vi "Find Minima and Walls.vi"() -> (3 "Low Points":cluster{i32, i32}[](array[cluster]), 5 "Wall":bool[][](array[boolean]))   [LabVIEW 2020]
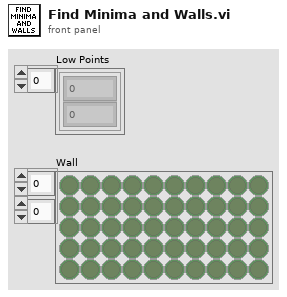
[diagram p1: front panel]
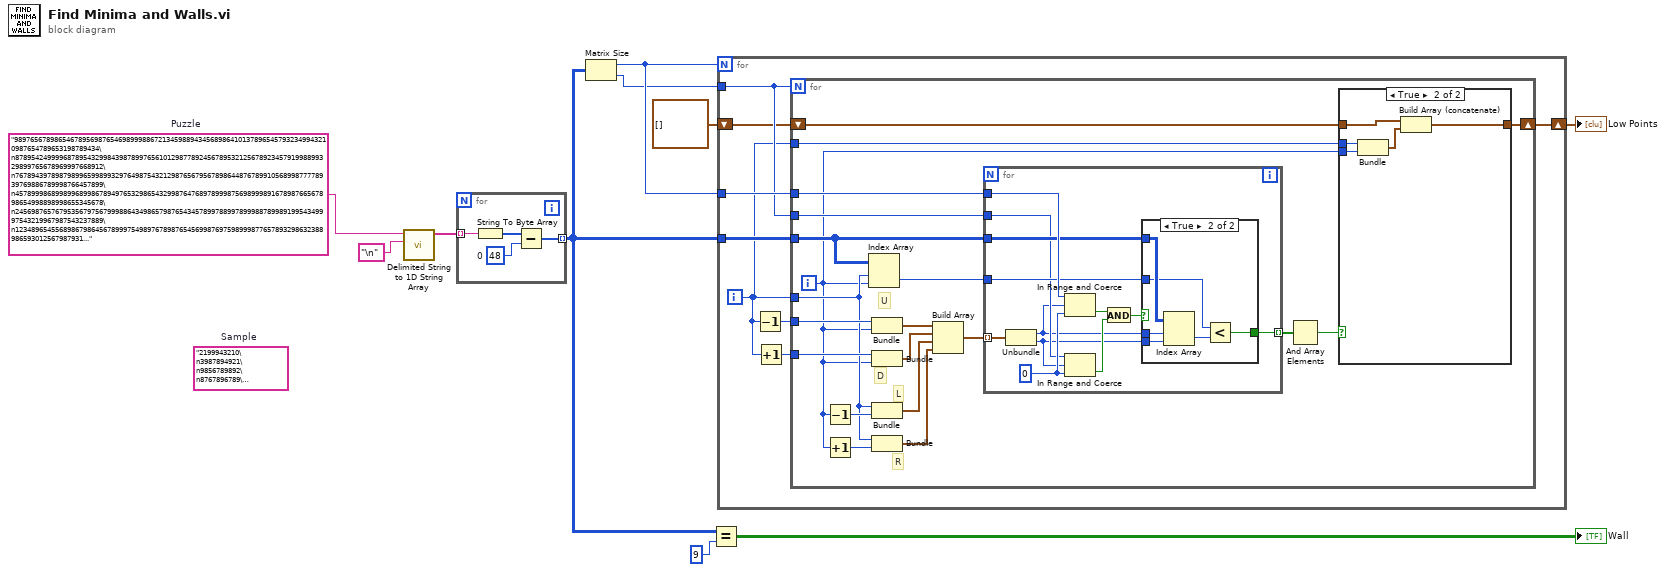
[diagram p0: block diagram]
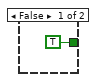
[diagram p3: hidden frame]
diagram:
  (unwired) "2199943210\n3987894921\n9856789892\n8767896789\n9899965678"  # Sample
  w1 = "9897656789865467895698765469899988672134598894345689864101378965457932349943210987654789653198789434\n8789542499996878954329984398789976561012987789245678953212567892345791998899329899765678969997668912\n7678943978987989965998993297649875432129876567956789864487678991056899877778939769886789998766457899\n4578999868998996899867894976532986543299876476897899987569899989167898766567898654998898998655345678\n2456987657679535679756799988643498657987654345789978899789998878998919954349997543219967987543237889\n12348965455689867986456789997549897678987654569987697598999877657893298632388986593012567987931..."  # Puzzle
  n1 = call <vilib>:"Delimited String to 1D String Array.vi"("delimiter"="\n", "delimited string"=w1) -> ("string array"=w9:string[])  [unwired: 9 in]
  n2 = for {
    tunnel: w9 -> [w14] mode=indexing
    tunnel: [w11] -> w4 mode=indexing
    w12 = u8 48  # 0
    n3 = String To Byte Array(string=w14) -> (unsigned byte array=w13:u8[])
    n4 = Subtract(x=w13, y=w12) -> (x-y=w11:u8[])
  }
  n5 = Matrix Size(0:w4) -> (1:w8:i32, 2:w7:i32)
  n6 = Equal?(x=w4, y=u8 9) -> (x = y?=→"Wall":bool[][])
  n7 = for {
    N: w8 -> [_]
    tunnel: w7 -> [w18]
    tunnel: w4 -> [w22]
    tunnel: w8 -> [w19]
    shift-right: [w16] -> w5
    shift-left: cluster{i32, i32}[] [] -> [w15]
    i -> [w17]
    n8 = Decrement(x=w17) -> (x-1=w21:i32)
    n9 = Increment(x=w17) -> (x+1=w20:i32)
    n10 = for {
      N: w18 -> [_]
      tunnel: w22 -> [w30]
      tunnel: w17 -> [w34]
      tunnel: w21 -> [w42]
      tunnel: w20 -> [w41]
      tunnel: w19 -> [w32]
      tunnel: w18 -> [w31]
      tunnel: w17 -> [w25]
      shift-right: [w24] -> w16
      shift-left: w15 -> [w23]
      i -> [w26]
      # "R"
      # "L"
      # "D"
      # "U"
      n11 = Decrement(x=w26) -> (x-1=w40:i32)
      n12 = Increment(x=w26) -> (x+1=w39:i32)
      n13 = Index Array(array=w30, index (row)=w34, index (col)=w26) -> (element=w27:u8)
      n14 = Bundle(w42, w26) -> (w38:cluster{i32, i32})  [unwired: 1 in]
      n15 = Bundle(w41, w26) -> (w37:cluster{i32, i32})  [unwired: 1 in]
      n16 = Bundle(w34, w40) -> (w36:cluster{i32, i32})  [unwired: 1 in]
      n17 = Bundle(w34, w39) -> (w35:cluster{i32, i32})  [unwired: 1 in]
      n18 = Build Array(w38, w37, w36, w35) -> (w33:cluster{i32, i32}[])
      n19 = for {
        tunnel: w33 -> [w60] mode=indexing
        tunnel: w32 -> [w59]
        tunnel: w31 -> [w52]
        tunnel: w27 -> [w55]
        tunnel: w30 -> [w54]
        tunnel: [w49] -> w29 mode=indexing
        w58 = 0 ("lower limit")
        n20 = Unbundle(w60) -> (w51:i32, w50:i32)
        n21 = In Range and Coerce(upper limit=w59, x=w51, lower limit=w58) -> (In Range?=w57:bool)  [unwired: 1 out]
        n22 = In Range and Coerce(upper limit=w52, x=w50, lower limit=w58) -> (In Range?=w56:bool)  [unwired: 1 out]
        n23 = And(x=w57, y=w56) -> (x .and. y?=w53:bool)
        n24 = case shown="True" w53 {
          tunnel: w55 -> [_ w64]
          tunnel: w54 -> [_ w67]
          tunnel: w51 -> [_ w66]
          tunnel: w50 -> [_ w65]
          tunnel: [TRUE w62] -> w49
          frame False {
          }
          frame True {
            n25 = Index Array(array=w67, index (row)=w66, index (col)=w65) -> (element=w63:u8)
            n26 = Less?(x=w64, y=w63) -> (x < y?=w62:bool)
          }
        }
      }
      n27 = And Array Elements(Boolean array=w29) -> (logical AND=w28:bool)
      n28 = case shown="True" w28 {
        tunnel: w26 -> [_ w48]
        tunnel: w25 -> [_ w47]
        tunnel: [w43 w45] -> w24
        tunnel: w23 -> [w43 w44]
        frame False {
        }
        frame True {
          n29 = Bundle(w47, w48) -> (w46:cluster{i32, i32})  [unwired: 1 in]
          n30 = Build Array (concatenate)(w44, w46) -> (w45:cluster{i32, i32}[])
        }
      }
    }
  }
  "Low Points" <- w5
